vi "Machine a etat led.vi"() -> ()   [LabVIEW 2017]
panel:
  in  "Stop":bool
  in  "loop":bool
  out "Boolean":bool
  in  "Blicking Time":dbl(slide) scale=0.5..2.0
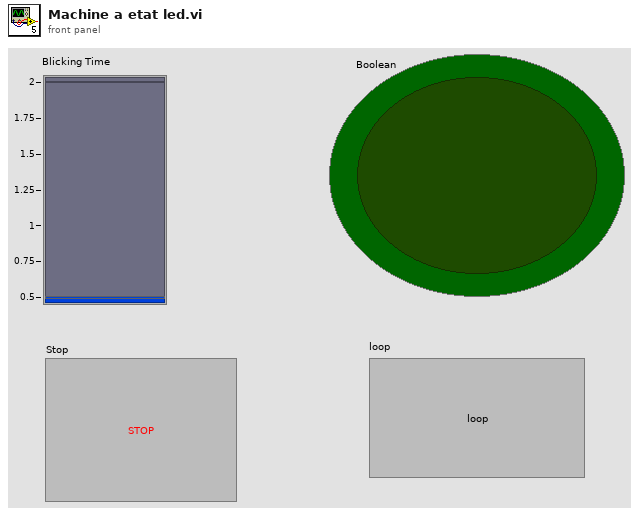
[diagram p1: front panel]
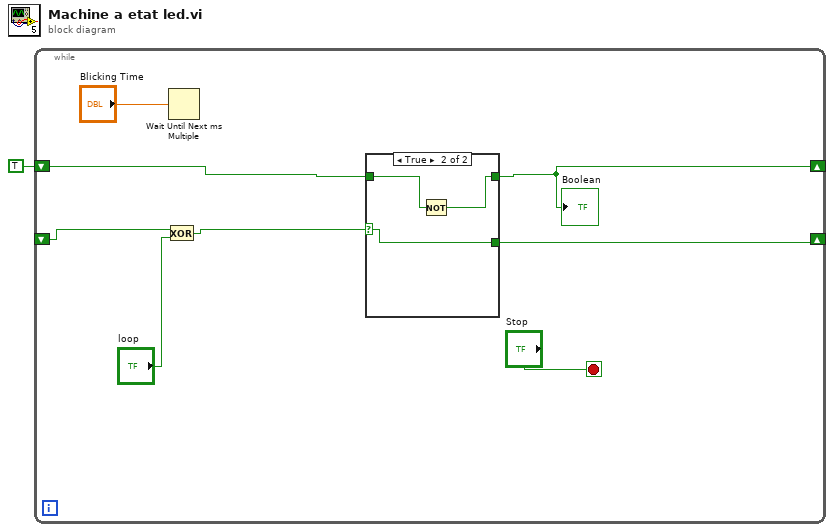
[diagram p0: block diagram]
diagram:
  n1 = while {
    shift-right: [w7] -> _
    shift-left: TRUE -> [w6]
    shift-right: [w5] -> _
    shift-left: _ -> [w4]
    stop <- "Stop" stop-if-true
    n2 = Exclusive Or(1:"loop", 2:w4) -> (0:w2:bool)
    n3 = Wait Until Next ms Multiple(millisecond multiple="Blicking Time") -> ()  [unwired: 1 out]
    n4 = case shown="True" w2 {
      selector: w2 -> [w10 w12]
      tunnel: [w11 w13] -> w7
      tunnel: w6 -> [w11 w14]
      tunnel: [w10 w12] -> w5
      frame False {
      }
      frame True {
        n5 = Not(x=w14) -> (.not. x?=w13:bool)
      }
    }
    "Boolean" <- w7
  }
